vi "Rear Rocket to Score.vi"() -> (4 "path":cluster{"X":dbl, "Y":dbl}[](array[cluster])=[{"X"=300.0, "Y"=62.0}, {"X"=299.67461844989043, "Y"=61.0694744519025}, {"X"=299.3484402711222, "Y"=60.139996027945}, {"X"=299.0206601828627, "Y"=59.212686491401676}, {"X"=298.6903421658294, "Y"=58.28878985895122}, {"X"=298.35640341524584, "Y"=57.36971426421218}, {"X"=298.017588735468, "Y"=56.45710738551117}, {"X"=297.6724059189975, "Y"=55.552961480396114}, {"X"=297.3190321299183, "Y"=54.65972826101114}, {"X"=296.9552059354967, "Y"=53.78044231811789}, {"X"=296.5781045689367, "Y"=52.91886589504286}, {"X"=296.1842067089792, "Y"=52.079694475910095}, {"X"=295.7690902080576, "Y"=51.26876688999192}, {"X"=295.3272603373312, "Y"=50.4934662515366}, {"X"=294.8517596590764, "Y"=49.76298229407969}, {"X"=294.3339218131716, "Y"=49.088921267233616}, {"X"=293.7490279537499, "Y"=48.443576558668006}, {"X"=293.11078706929555, "Y"=47.82106577294344}, {"X"=292.43011553227353, "Y"=47.21671181213899}, {"X"=291.7157011841359, "Y"=46.626804386429704}, {"X"=290.9744453098971, "Y"=46.04839097291032}, {"X"=290.21183273049894, "Y"=45.479116467940116}, {"X"=289.43223242124526, "Y"=44.91710715247492}, {"X"=288.63912719749015, "Y"=44.36087877327859}, {"X"=287.8352882443134, "Y"=43.80925637821033}, {"X"=287.02291524353586, "Y"=43.26130609055709}, {"X"=286.2037537147513, "Y"=42.716282319122264}, {"X"=285.3791917054477, "Y"=42.17358975864675}, {"X"=284.55033575832124, "Y"=41.63275547592639}, {"X"=283.71806878273304, "Y"=41.09340621831047}, {"X"=282.8830947765157, "Y"=40.55524861604157}, {"X"=282.0459749214442, "Y"=40.01805232919511}, {"X"=281.20715746642963, "Y"=39.48163687452977}, {"X"=280.36700205234155, "Y"=38.9458621800215}, {"X"=279.52579871138164, "Y"=38.41062199981987}, {"X"=278.6837823205853, "Y"=37.875839008144894}, {"X"=277.8411438825949, "Y"=37.34146076340328}, {"X"=276.9980400380976, "Y"=36.80745637726766}, {"X"=276.1546016901654, "Y"=36.27381417913622}, {"X"=275.31094194564014, "Y"=35.74054073741807}, {"X"=274.4671631625032, "Y"=35.207661380817036}, {"X"=273.623362892874, "Y"=34.675222091527786}, {"X"=272.77963881439433, "Y"=34.143292517837864}, {"X"=271.9360931036315, "Y"=33.611969942692625}, {"X"=271.0928369175939, "Y"=33.081384286885545}, {"X"=270.249995642004, "Y"=32.551704502682924}, {"X"=269.407715399353, "Y"=32.023146926770664}, {"X"=268.5661711147921, "Y"=31.495986274378406}, {"X"=267.7255763318321, "Y"=30.97056999819698}, {"X"=266.88619501114016, "Y"=30.447336772700634}, {"X"=266.048355725766, "Y"=29.92683996561209}, {"X"=265.2124689337283, "Y"=29.409777169871585}, {"X"=264.3790483081579, "Y"=28.897027209260248}, {"X"=263.54873734699845, "Y"=28.389696460153502}, {"X"=262.7223433889556, "Y"=27.889177277174706}, {"X"=261.90087674370676, "Y"=27.397219197488017}, {"X"=261.08561804553267, "Y"=26.916028809903498}, {"X"=260.2781408719905, "Y"=26.448361127366653}, {"X"=259.4804970761633, "Y"=25.997717949132273}, {"X"=258.6951597539513, "Y"=25.568451149135008}, {"X"=257.9253315190208, "Y"=25.166069056782653}, {"X"=257.13530610127395, "Y"=24.772438639305566}, {"X"=256.3330206988861, "Y"=24.384619056087708}, {"X"=255.5257731958763, "Y"=24.0}])   [LabVIEW 2018]
uses:
  AutonBuilder/Typedef/Data Point.ctl
panel:
  in  "Data Points":T1[](array[typedef])=[{"X"=300.0, "Y"=62.0, "Theta"=0.0, "Speed %"=0.0, "Disabled?"=FALSE}, {"X"=295.60824742268045, "Y"=48.54355400696864, "Theta"=0.0, "Speed %"=0.0, "Disabled?"=FALSE}, {"X"=258.30927835051546, "Y"=25.0, "Theta"=0.0, "Speed %"=0.0, "Disabled?"=FALSE}, {"X"=255.5257731958763, "Y"=24.0, "Theta"=0.0, "Speed %"=0.0, "Disabled?"=FALSE}]
  out "Graph":cluster{dbl[], dbl[]}[](graph)=[{[0.0, 33.5, 33.5, 0.0, 0.0], [126.25, 126.25, 97.75, 97.75, 126.25]}, {[300.0, 295.60824742268045, 258.30927835051546, 255.5257731958763], [62.0, 48.54355400696864, 25.0, 24.0]}, {[300.0, 299.67461844989043, 299.3484402711222, 299.0206601828627, 298.6903421658294, 298.35640341524584, 298.017588735468, 297.6724059189975, 297.3190321299183, 296.9552059354967, 296.5781045689367, 296.1842067089792, 295.7690902080576, 295.3272603373312, 294.8517596590764, 294.3339218131716, 293.7490279537499, 293.11078706929555, 292.43011553227353, 291.7157011841359, 290.9744453098971, 290.21183273049894, 289.43223242124526, 288.63912719749015, 287.8352882443134, 287.02291524353586, 286.2037537147513, 285.3791917054477, 284.55033575832124, 283.71806878273304, 282.8830947765157, 282.0459749214442, 281.20715746642963, 280.36700205234155, 279.52579871138164, 278.6837823205853, 277.8411438825949, 276.9980400380976, 276.1546016901654, 275.31094194564014, 274.4671631625032, 273.623362892874, 272.77963881439433, 271.9360931036315, 271.0928369175939, 270.249995642004, 269.407715399353, 268.5661711147921, 267.7255763318321, 266.88619501114016, 266.048355725766, 265.2124689337283, 264.3790483081579, 263.54873734699845, 262.7223433889556, 261.90087674370676, 261.08561804553267, 260.2781408719905, 259.4804970761633, 258.6951597539513, 257.9253315190208, 257.13530610127395, 256.3330206988861, 255.5257731958763], [62.0, 61.0694744519025, 60.139996027945, 59.212686491401676, 58.28878985895122, 57.36971426421218, 56.45710738551117, 55.552961480396114, 54.65972826101114, 53.78044231811789, 52.91886589504286, 52.079694475910095, 51.26876688999192, 50.4934662515366, 49.76298229407969, 49.088921267233616, 48.443576558668006, 47.82106577294344, 47.21671181213899, 46.626804386429704, 46.04839097291032, 45.479116467940116, 44.91710715247492, 44.36087877327859, 43.80925637821033, 43.26130609055709, 42.716282319122264, 42.17358975864675, 41.63275547592639, 41.09340621831047, 40.55524861604157, 40.01805232919511, 39.48163687452977, 38.9458621800215, 38.41062199981987, 37.875839008144894, 37.34146076340328, 36.80745637726766, 36.27381417913622, 35.74054073741807, 35.207661380817036, 34.675222091527786, 34.143292517837864, 33.611969942692625, 33.081384286885545, 32.551704502682924, 32.023146926770664, 31.495986274378406, 30.97056999819698, 30.447336772700634, 29.92683996561209, 29.409777169871585, 28.897027209260248, 28.389696460153502, 27.889177277174706, 27.397219197488017, 26.916028809903498, 26.448361127366653, 25.997717949132273, 25.568451149135008, 25.166069056782653, 24.772438639305566, 24.384619056087708, 24.0]}, {[302.86477858502263, 286.22327445702683, 285.90234571545136, 285.5852974223649, 285.2721534701492, 284.9630813103694, 284.65854491497066, 284.3596146890509, 284.0682845244903, 283.7878800239722, 283.5237622881228, 283.284586590675, 283.0844706153398, 282.94655571314365, 282.9090663187071, 283.0335988010247, 283.1903727320916, 283.1610090907952, 282.9689438463796, 282.6425263719427, 282.20803895179876, 281.6875849481578, 281.09908429726573, 280.4568791466025, 279.7723485422993, 279.05443856021975, 278.31014735286635, 277.54496481222986, 276.7632314491956, 275.96839879288314, 275.16320977810483, 274.3498342602443, 273.5299854983688, 272.705024324649, 271.87604559543666, 271.04394160612594, 270.2094442912699, 269.37315433050924, 268.5355663072881, 267.6970953497151, 266.858105591195, 266.0189375374354, 265.1799312743281, 264.34144462601915, 263.5038681236345, 262.66764045359264, 261.8332683295524, 261.0013538316898, 260.1726310562781, 259.3480132875298, 258.5286523694241, 257.716013646025, 256.9119726705063, 256.1189438006737, 255.3400569425504, 254.57940304713003, 253.84240041308206, 253.13630509062725, 252.4710267873329, 251.8604635934824, 251.3243213621097, 250.7803716505439, 250.1312411066753, 249.396420590183], [48.0409332812399, 65.77307358295656, 64.85858068862031, 63.96174192315117, 63.08615498234137, 62.23607049809267, 61.41678965376509, 60.635489362056504, 59.90188315163048, 59.22874740683094, 58.63259039096977, 58.134634674082335, 57.76206541909399, 57.54900684093302, 57.53695012125133, 57.77023452164063, 58.01317947154524, 58.022262672256225, 57.87263647075209, 57.61497979581334, 57.28282996934859, 56.898385259997326, 56.476568313957166, 56.02763997053232, 55.55878842683612, 55.0751064675504, 54.58023944158393, 54.07684095256779, 53.566887471123884, 53.051880830417986, 52.53297275760165, 52.011046906156494, 51.48678287834082, 50.96071121362751, 50.433258036275866, 49.90477636178045, 49.375564857508905, 48.84587894611838, 48.3159402303974, 47.78594816156611, 47.25609459333546, 46.72657948451729, 46.197625568880554, 45.669491018830165, 45.142480946987, 44.61695998264567, 44.09336861432842, 43.57224560718824, 43.054258080255636, 42.540240324032986, 42.03124252966374, 41.52859139072113, 41.03396592631697, 40.54949365661164, 40.077874780321714, 39.62254221613808, 39.187878643117585, 38.779487664388306, 38.404563892804006, 38.072427652394744, 37.79497102442642, 37.526940124151, 37.21428896180382, 36.86442912200463]}, {[297.13522141497737, 313.12596244275403, 312.794534826793, 312.4560229433605, 312.1085308615096, 311.7497255201223, 311.37663255596533, 310.98519714894417, 310.5697797353463, 310.12253184702115, 309.6324468497506, 309.0838268272834, 308.4537098007754, 307.70796496151877, 306.79445299944564, 305.63424482531855, 304.30768317540816, 303.06056504779593, 301.89128721816746, 300.7888759963291, 299.7408516679954, 298.7360805128401, 297.7653805452248, 296.8213752483778, 295.8982279463275, 294.991391926852, 294.0973600766363, 293.2134185986655, 292.3374400674469, 291.46773877258295, 290.60297977492655, 289.74211558264415, 288.8843294344905, 288.0289797800341, 287.1755518273266, 286.32362303504465, 285.4728434739199, 284.62292574568596, 283.7736370730427, 282.9247885415652, 282.0762207338114, 281.2277882483126, 280.37934635446055, 279.53074158124383, 278.6818057115533, 277.8323508304154, 276.98216246915354, 276.1309883978944, 275.2785216073861, 274.4243767347505, 273.5680590821079, 272.70892422143163, 271.8461239458095, 270.9785308933232, 270.1046298353608, 269.2223504402835, 268.32883567798325, 267.41997665335373, 266.48996736499373, 265.52985591442024, 264.5263416759319, 263.490240552004, 262.53480029109693, 261.65512580156957], [75.9590667187601, 56.365875320848446, 55.4214113672697, 54.46363105965218, 53.49142473556107, 52.50335803033168, 51.49742511725725, 50.470433598735724, 49.4175733703918, 48.33213722940484, 47.20514139911596, 46.024754277737856, 44.77546836088985, 43.43792566214019, 41.98901446690805, 40.4076080128266, 38.87397364579077, 37.61986887363066, 36.56078715352589, 35.63862897704607, 34.81395197647205, 34.05984767588291, 33.35764599099267, 32.694117576024865, 32.05972432958454, 31.44750571356379, 30.8523251966606, 30.270338564725705, 29.69862348072889, 29.134931606202954, 28.577524474481486, 28.02505775223372, 27.47649087071872, 26.931013146415488, 26.387985963363867, 25.846901654509335, 25.30735666929766, 24.769033808416943, 24.231688127875028, 23.695133313270034, 23.15922816829861, 22.623864698538284, 22.08895946679517, 21.554448866555084, 21.02028762678409, 20.486449022720176, 19.95292523921291, 19.41972694156857, 18.88688191613832, 18.354433221368282, 17.82243740156044, 17.290962949022035, 16.76008849220353, 16.229899263695366, 15.700479774027697, 15.171896178837956, 14.644178976689409, 14.117234590345, 13.590872005460536, 13.06447464587527, 12.537167089138887, 12.017937154460135, 11.554949150371597, 11.135570877995368]}, {[], []}, {[], []}, {[], []}, {[], []}, {[], []}, {[], []}, {[], []}, {[], []}, {[], []}, {[], []}, {[], []}, {[], []}, {[], []}, {[], []}, {[], []}, {[], []}, {[], []}, {[], []}, {[], []}, {[], []}]
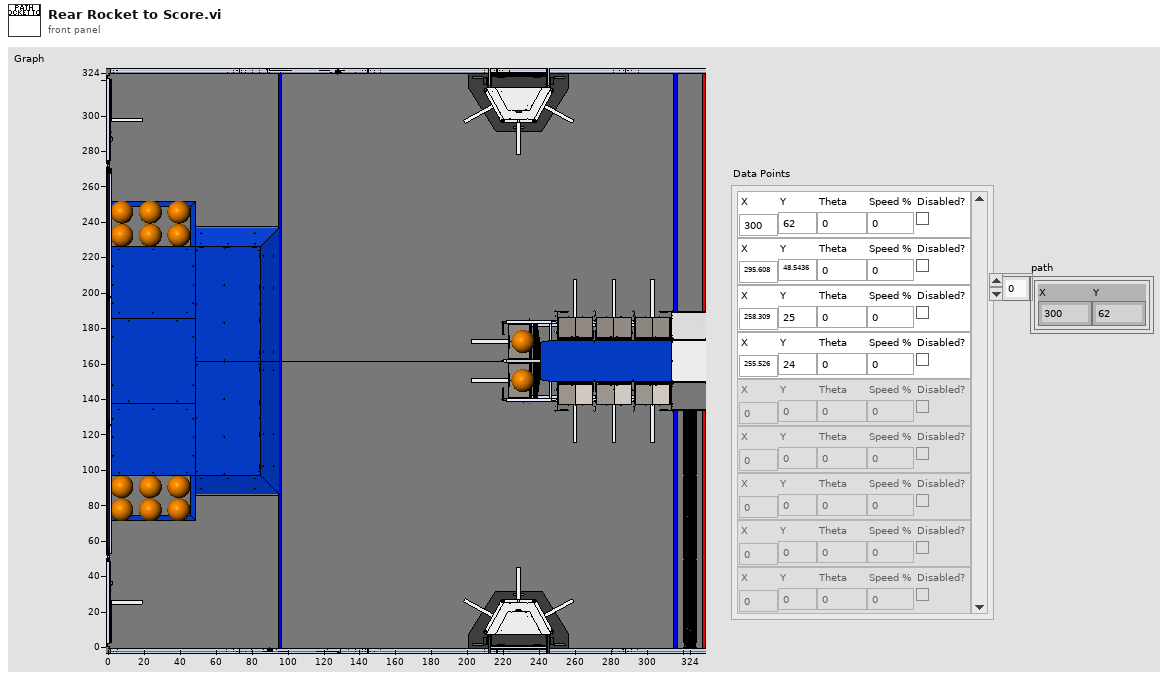
[diagram p1: front panel]
types:
  T1 = typedef "Data Point.ctl" = cluster{"X":dbl, "Y":dbl, "Theta":dbl, "Speed %":dbl, "Disabled?":bool}
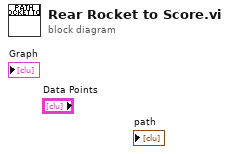
[diagram p0: block diagram]
diagram:
